vi "Undistort (ARGB).vi"(6 "Camera Parameters":T1, 8 "error in (no error)":errorcluster, 10 "ARGB Image Destination in":T4, 11 "ARGB Image Source in":T4) -> (0 "error out":errorcluster, 3 "ARGB Image Destination":T4)   [LabVIEW 2020, in "image.lvlib"]
doc: "Undistorts the Source image to correct for the Distortion values on the Camera Parameters.\n\nIf more control over the undistortion process is required or if the same Distortion needs to be corrected in multiple images then use the \"Image Undistorter.lvclass\" to avoid duplicate calculations."
uses:
  image.lvlib
  ARGB Image.ctl
  common/Camera Parameters.ctl
  common/Camera Matrix.ctl
  common/Camera Distortion Coefficients.ctl
  88690800-d834-48c3-9c45-44dd73aae051.vi
  <vilib>/Utility/error.llb/Error Cluster From Error Code.vi
  common/common.lvlib
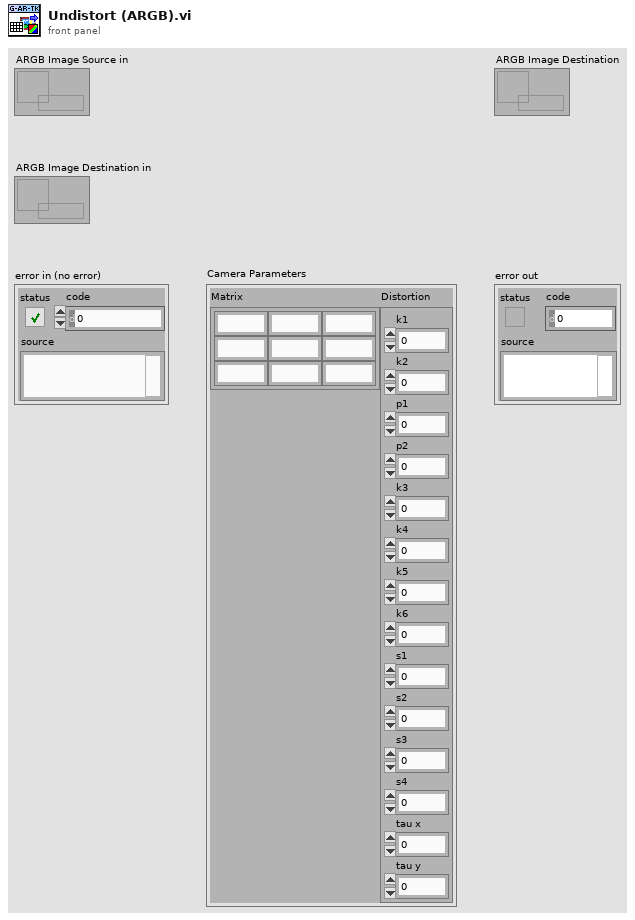
[diagram p1: front panel]
types:
  T1 = typedef "common.lvlib/Camera Parameters.ctl" = cluster{"Matrix":T2, "Distortion":T3}
  T2 = typedef "common.lvlib/Camera Matrix.ctl" = cluster{"m 0,0":dbl, "m 0,1":dbl, "m 0,2":dbl, "m 1,0":dbl, "m 1,1":dbl, "m 1,2":dbl, "m 2,0":dbl, "m 2,1":dbl, "m 2,2":dbl}
  T3 = typedef "common.lvlib/Camera Distortion Coefficients.ctl" = cluster{"k1":dbl, "k2":dbl, "p1":dbl, "p2":dbl, "k3":dbl, "k4":dbl, "k5":dbl, "k6":dbl, "s1":dbl, "s2":dbl, "s3":dbl, "s4":dbl, "tau x":dbl, "tau y":dbl}
  T4 = typedef "image.lvlib/ARGB Image.ctl" = refnum<data-value>
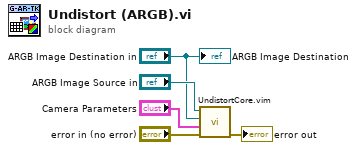
[diagram p0: block diagram]
diagram:
  n1 = call "UndistortCore.vim"("error in (no error)"="error in (no error)", "Camera Parameters"="Camera Parameters", "Dst"="ARGB Image Destination in", "Src"="ARGB Image Source in") -> ("error out"=→"error out":errorcluster)  [unwired: 7 in]
  "ARGB Image Destination" <- "ARGB Image Destination in"
